vi "client.vi"(7 "Tab Control":enum32{"Check Connexion", "Post"}(tab)=enum."Post", 10 "File Path Image":path, 11 "url post":string="http://localhost:8501/v1/models/resnet:predict") -> (3 "body":string)   [LabVIEW 2018]
uses:
  <vilib>/httpClient/POSTBuffer.vi
  <vilib>/httpClient/LabVIEWHTTPClient.lvlib
panel:
  in  "url Check":string="http://localhost:8501/v1/models/resnet"
  out "body get respons":string
  out "headers get respons":string="\r\n\r\n"
  in  "timeout (10000)":i32=10000
  out "headers":string="\r\n"
  out "resulting reading string":string
  out "error out":errorcluster
  in  "error in (no error)":errorcluster
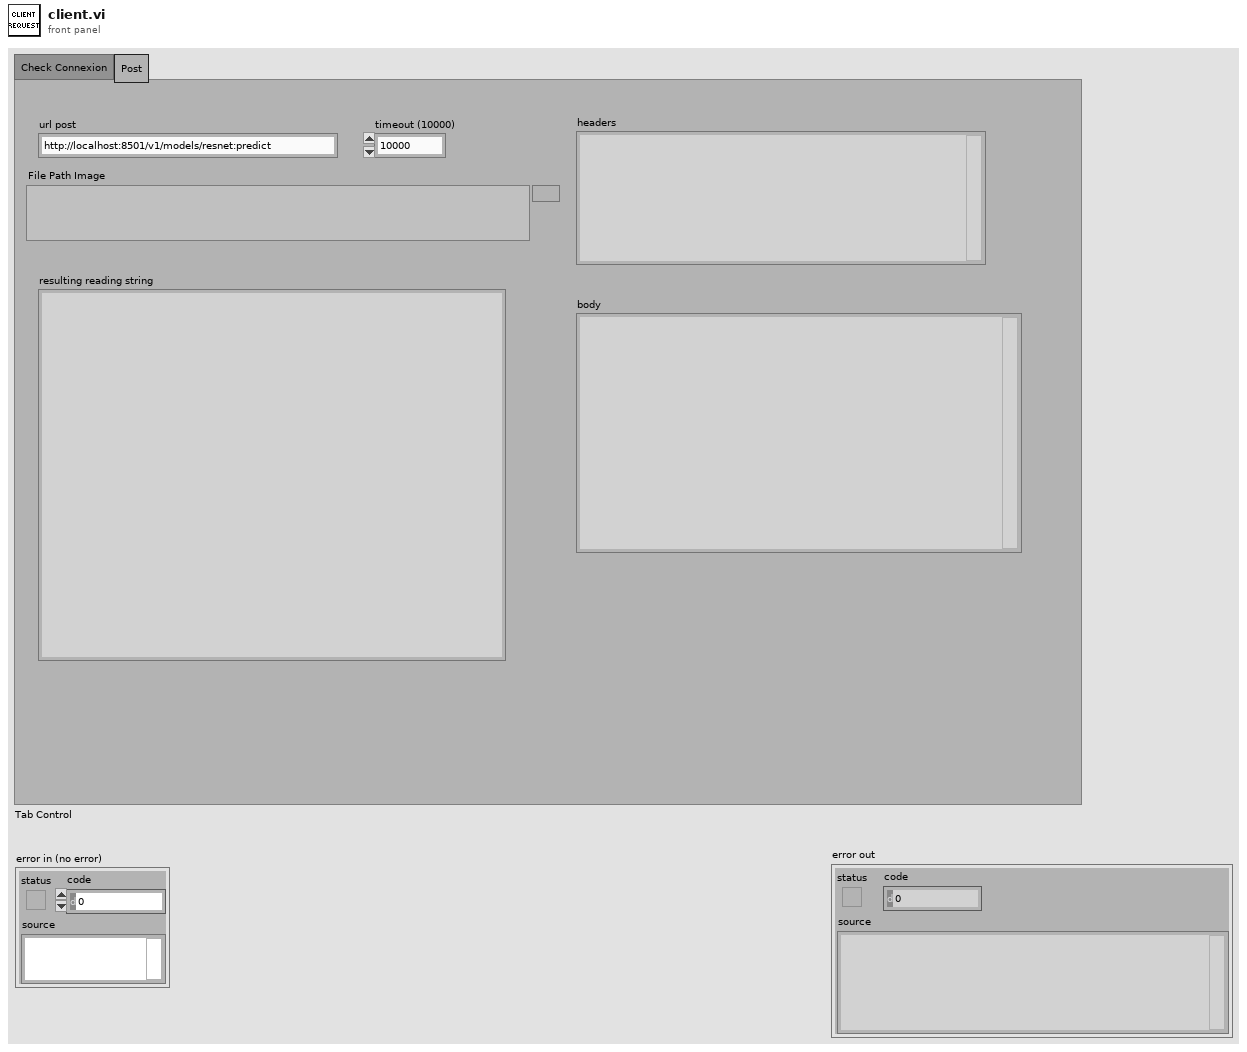
[diagram p1: front panel]
types:
  T1 = typedef "LabVIEWHTTPClient.lvlib/ClientHandle.ctl" = refnum<k1>
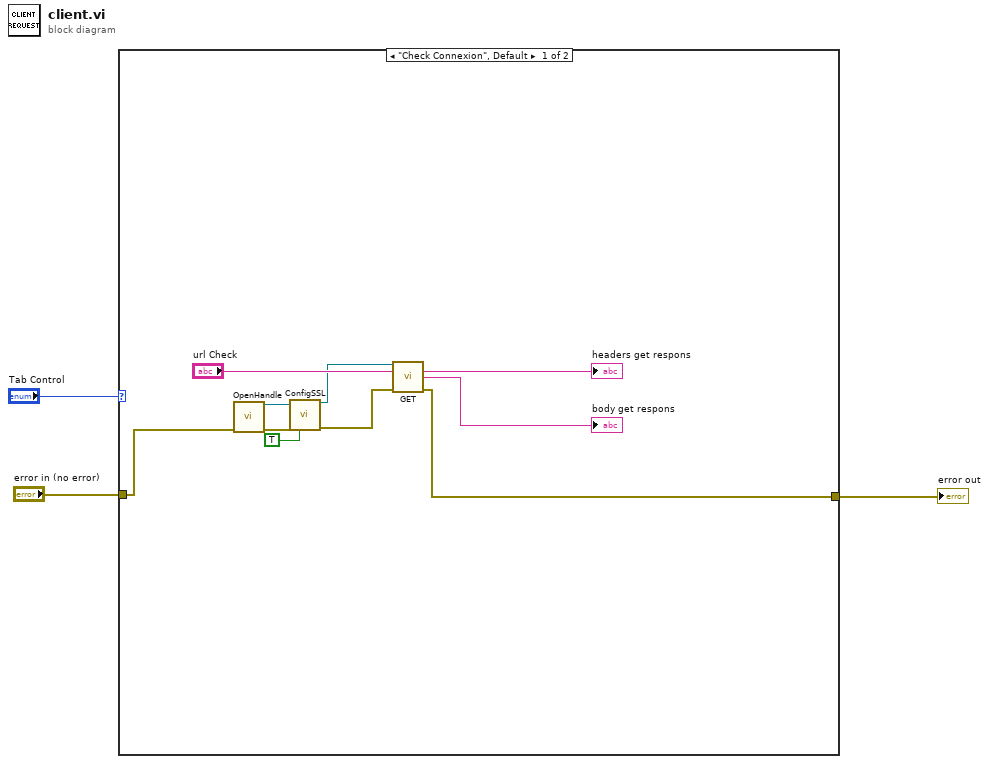
[diagram p0: block diagram]
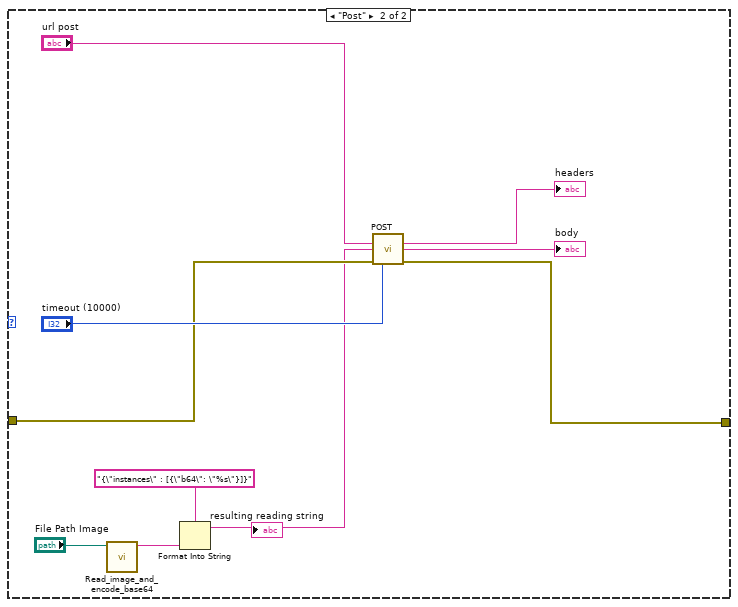
[diagram p2: hidden frame]
diagram:
  n1 = case shown="\"Check Connexion\", Default" "Tab Control" {
    tunnel: "error in (no error)" -> [w4 w19]
    tunnel: [w10 w18] -> w1
    frame "Check Connexion", Default {
      n2 = call <vilib>:"OpenHandle.vi"("error in (no error)"=w4) -> ("client handle out"=w7:T1, "error out"=w6:errorcluster)  [unwired: 13 in]
      n3 = call <vilib>:"ConfigSSL.vi"("client handle"=w7, "error in (no error)"=w6, "verify server (true)"=TRUE) -> ("client handle out"=w9:T1, "error out"=w5:errorcluster)  [unwired: 11 in]
      n4 = call <vilib>:"GET.vi"("client handle"=w9, "url"="url Check", "error in (no error)"=w5) -> ("headers"=→"headers get respons":string, "body"=→"body get respons":string, "error out"=w10:errorcluster)  [unwired: 9 in, 1 out]
    }
    frame "Post" {
      n5 = call "Read_image_and_encode_base64.vi"("File Path"="File Path Image") -> ("Base64 String"=w14:string)  [unwired: 10 in]
      n6 = Format Into String(format string="{\"instances\" : [{\"b64\": \"%s\"}]}", w14) -> (resulting string=w15:string)  [unwired: 2 in, 1 out]
      "resulting reading string" <- w15
      n7 = call-poly <vilib>:"POST.vi"("url"="url post", "buffer"=w15, "error in (no error)"=w19, "timeout (10000)"="timeout (10000)") -> ("headers"=→"headers":string, "body"=→"body":string, "error out"=w18:errorcluster)  [unwired: 8 in, 1 out]
    }
  }
  "error out" <- w1
